vi "Query.vi"(8 "error in (no error)":errorcluster caption="entrée d'erreur (pas d'erreur)", 11 "Database Drivers en entrée":refnum<class "Database Drivers.lvclass">) -> (0 "error out":errorcluster caption="sortie d'erreur", 3 "Database Drivers en sortie":refnum<class "Database Drivers.lvclass">)   [LabVIEW 2020, in "Library Instrument & Equipement.lvlib" / "Library Database.lvlib" / "Database Drivers.lvclass"]
uses:
  Database Drivers.lvclass
  <vilib>/addons/database/Connection.llb/Conn Execute.vi
  <vilib>/addons/database/Recordset.llb/Rec Fetch Recordset Data (R).vi
  <vilib>/addons/database/Recordset.llb/Rec Destroy - Connection.vi
  Database Drivers.lvclass/Database Drivers.ctl
  <vilib>/addons/database/NI_Database_API.lvlib
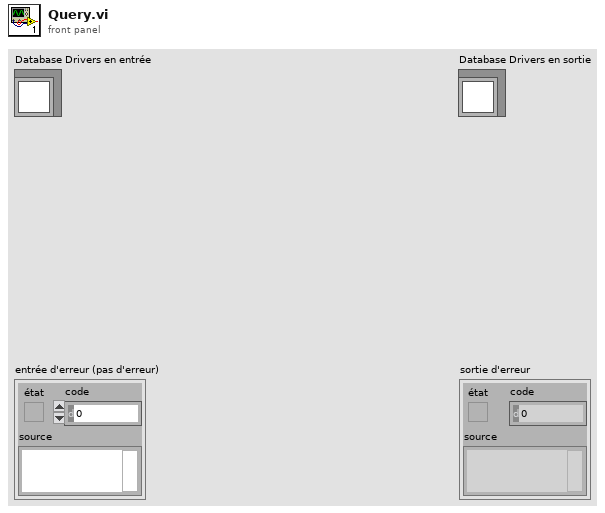
[diagram p1: front panel]
types:
  T1 = typedef "NI_Database_API.lvlib/Conn ObjectReference.ctl" = refnum<k1>
  T2 = typedef "NI_Database_API.lvlib/Rec ObjectReference.ctl" = refnum<k1>
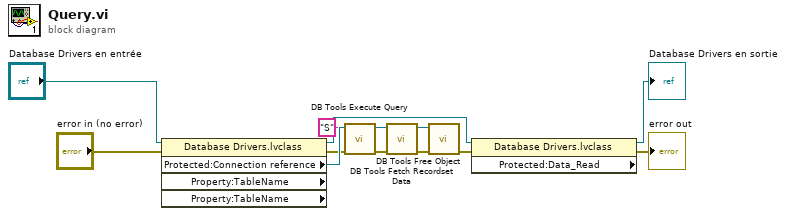
[diagram p0: block diagram]
diagram:
  n1 = property class="Database Drivers.lvclass" props=["Protected:Connection reference", "Property:TableName", "Property:TableName"](reference="Database Drivers en entrée", error in="error in (no error)") -> (reference out=w6:refnum<class "Database Drivers.lvclass">, error out=w5:errorcluster, "Protected:Connection reference"=w7:T1)  [unwired: 2 out]
  n2 = call-poly <vilib>:"DB Tools Execute Query.vi"("error in (no error)"=w5, "SQL query"="S", "connection reference"=w7) -> ("error out"=w9:errorcluster, "recordset reference"=w10:T2)  [unwired: 5 in]
  n3 = call-poly <vilib>:"DB Tools Fetch Recordset Data.vi"("error in (no error)"=w9, "recordset reference"=w10) -> ("error out"=w8:errorcluster, "recordset reference out"=w11:T2)  [unwired: 3 in, 1 out]
  n4 = call-poly <vilib>:"DB Tools Free Object.vi"("error in (no error)"=w8, "recordset reference"=w11) -> ("error out"=w4:errorcluster)  [unwired: 8 in, 1 out]
  n5 = property class="Database Drivers.lvclass" props=["Protected:Data_Read"](reference=w6, error in=w4) -> (reference out=→"Database Drivers en sortie":refnum<class "Database Drivers.lvclass">, error out=→"error out":errorcluster)  [unwired: 1 out]
